vi "Set value by Column.vi"(8 "error in (no error)":errorcluster, 10 "Value Column":refnum<class "Column Interface.lvclass">, 11 "Column in":refnum<class "Composed Column.lvclass">) -> (0 "error out":errorcluster, 3 "Column out":refnum<class "Composed Column.lvclass">)   [LabVIEW 2020, in "Composed Columns.lvlib" / "Composed Column.lvclass"]
uses:
  Composed Column.lvclass
  Column Interface/Column Interface Class/Column Interface.lvclass
  Composed Column.lvclass/Composed Column.ctl
  Basic Columns/Column Configuration/Basic Column Configuration Class/Column Configuration.lvclass
  Database Libraries/Database Interfaces/Database Interface Class/Database Interface.lvclass
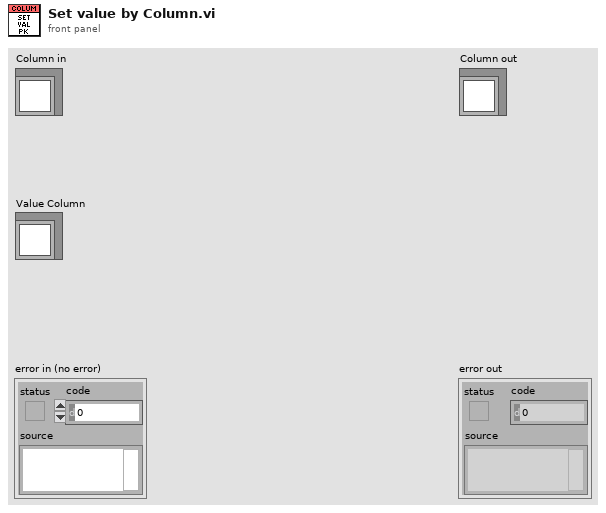
[diagram p1: front panel]
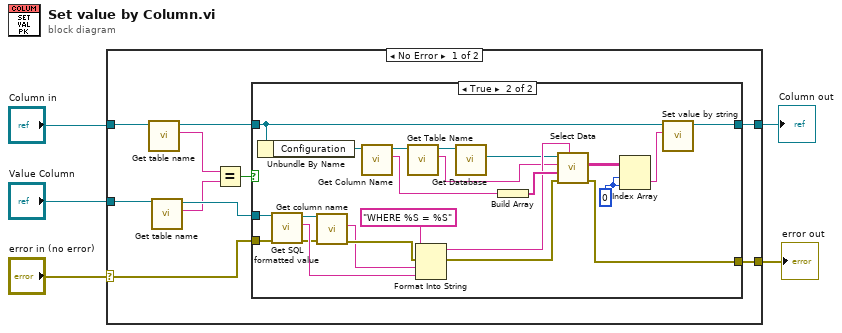
[diagram p0: block diagram]
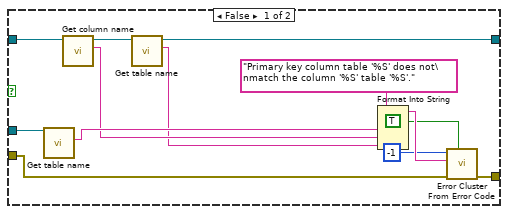
[diagram p2: hidden frame]
diagram:
  n1 = case shown="No Error" "error in (no error)" {
    selector: "error in (no error)" -> [w14 w53]
    tunnel: [w12 w53] -> w2
    tunnel: [w13 w52] -> w1
    tunnel: "Column in" -> [w7 w52]
    tunnel: "Value Column" -> [w11 _]
    frame No Error {
      n2 = call-dynamic "Get table name.vi"("Column in"=w7) -> ("Table Name"=w8:string, "Column out"=w6:refnum<class "Composed Column.lvclass">)  [unwired: 8 in, 1 out]
      n3 = call-dynamic "Get table name.vi"("Column Interface in"=w11) -> ("Table Name"=w9:string, "Column Interface out"=w10:refnum<class "Column Interface.lvclass">)  [unwired: 8 in, 1 out]
      n4 = Equal?(x=w8, y=w9) -> (x = y?=w15:bool)
      n5 = case shown="True" w15 {
        tunnel: w10 -> [w22 w49]
        tunnel: w6 -> [w20 w35]
        tunnel: w14 -> [w23 w46]
        tunnel: [w18 w37] -> w13
        tunnel: [w25 w40] -> w12
        frame False {
          n6 = call-dynamic "Get table name.vi"("Column Interface in"=w22) -> ("Table Name"=w21:string)  [unwired: 8 in, 2 out]
          n7 = call-dynamic "Get column name.vi"("Column in"=w20) -> ("Name"=w17:string, "Column out"=w19:refnum<class "Composed Column.lvclass">)  [unwired: 8 in, 1 out]
          n8 = call-dynamic "Get table name.vi"("Column in"=w19) -> ("Table Name"=w16:string, "Column out"=w18:refnum<class "Composed Column.lvclass">)  [unwired: 8 in, 1 out]
          n9 = Format Into String(format string="Primary key column table '%S' does not\nmatch the column '%S' table '%S'.", w21, w17, w16) -> (resulting string=w27:string)  [unwired: 2 in, 1 out]
          n10 = call <vilib>:"Error Cluster From Error Code.vi"("show call chain? (False)"=TRUE, "error in (no error)"=w23, "error message (\"\")"=w27, "error code (0)"=-1) -> ("error out"=w25:errorcluster)  [unwired: 5 in]
        }
        frame True {
          w41 = 0 ("index (row)")
          n11 = Unbundle By Name(w35) -> ("Configuration"=w34:refnum<class "Column Configuration.lvclass">)
          n12 = call-dynamic "Get SQL formatted value.vi"("error in (no error)"=w46, "Column Interface in"=w49) -> ("error out"=w45:errorcluster, "Formatted Value"=w50:string, "Column Interface out"=w48:refnum<class "Column Interface.lvclass">)  [unwired: 7 in]
          n13 = call-dynamic "Get column name.vi"("error in (no error)"=w45, "Column Interface in"=w48) -> ("error out"=w44:errorcluster, "Name"=w39:string)  [unwired: 7 in, 1 out]
          n14 = call-dynamic "Get Column Name.vi"("Basic Column Configuration in"=w34) -> ("Column Name"=w30:string, "Basic Column Configuration out"=w33:refnum<class "Column Configuration.lvclass">)  [unwired: 8 in, 1 out]
          n15 = call-dynamic "Get Table Name.vi"("Basic Column Configuration in"=w33) -> ("Table Name"=w29:string, "Basic Column Configuration out"=w32:refnum<class "Column Configuration.lvclass">)  [unwired: 8 in, 1 out]
          n16 = Format Into String(initial string="WHERE %S = %S", error in=w44, w39, w50) -> (resulting string=w36:string, error out=w43:errorcluster)  [unwired: 1 in]
          n17 = call-dynamic "Get Database.vi"("Basic Column Configuration in"=w32) -> ("Database"=w31:refnum<class "Database Interface.lvclass">)  [unwired: 8 in, 2 out]
          n18 = Build Array(w30) -> (w47:string[])
          n19 = call-dynamic "Select Data.vi"("WHERE Statement"=w36, "error in (no error)"=w43, "Columns"=w47, "Table"=w29, "Database Interface in"=w31) -> ("error out"=w40:errorcluster, "Data"=w42:string[][])  [unwired: 4 in, 1 out]
          n20 = Index Array(array=w42, index (row)=w41, index (col)=w41) -> (element=w38:string)
          n21 = call-dynamic "Set value by string.vi"("Value"=w38, "Column in"=w35) -> ("Column out"=w37:refnum<class "Composed Column.lvclass">)  [unwired: 8 in, 1 out]
        }
      }
    }
    frame Error {
    }
  }
  "error out" <- w2
  "Column out" <- w1
